vi "RunStatsForIndividualIpAddresses.vi"(8 "IpStatus (in)":T2[](array[typedef]) {"%rtk" scale=0.0..60.0; "TimePing" scale=0.0..60.0}, 11 "IP list (in)":T1) -> (0 "IpStatus(out)":T2[](array[typedef]) {"%rtk" scale=0.0..60.0; "TimePing" scale=0.0..60.0}, 3 "IP list (out)":T1)   [LabVIEW 2011]
uses:
  GPS String Capture Software/IP RTK status Indicator.ctl
  ArrayIpAddressesAndReportingCheckbox.ctl
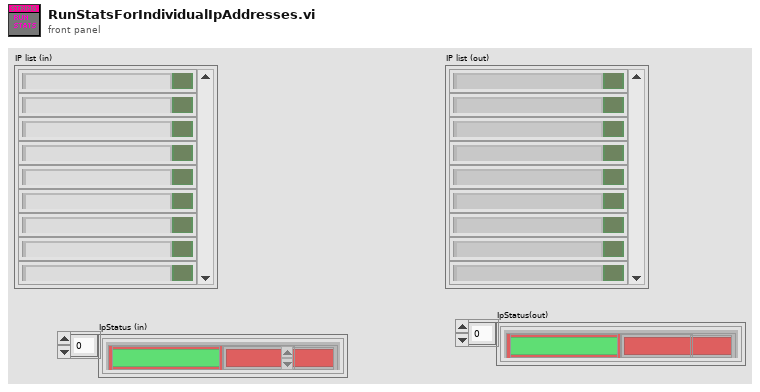
[diagram p1: front panel]
types:
  T1 = typedef "ArrayIpAddressesAndReportingCheckbox.ctl" = cluster{"IpAddress":string, "Report Errors":bool}[]
  T2 = typedef "IP RTK status Indicator.ctl" = cluster{"TimePing":dbl, "IP":string, "%rtk":dbl, "Lastrtk":string, "MinLastRTk":dbl, "RTK Count":bool[], "Last Nema Time":dbl, "Last RTK Time":dbl, "Last Ping time":dbl}
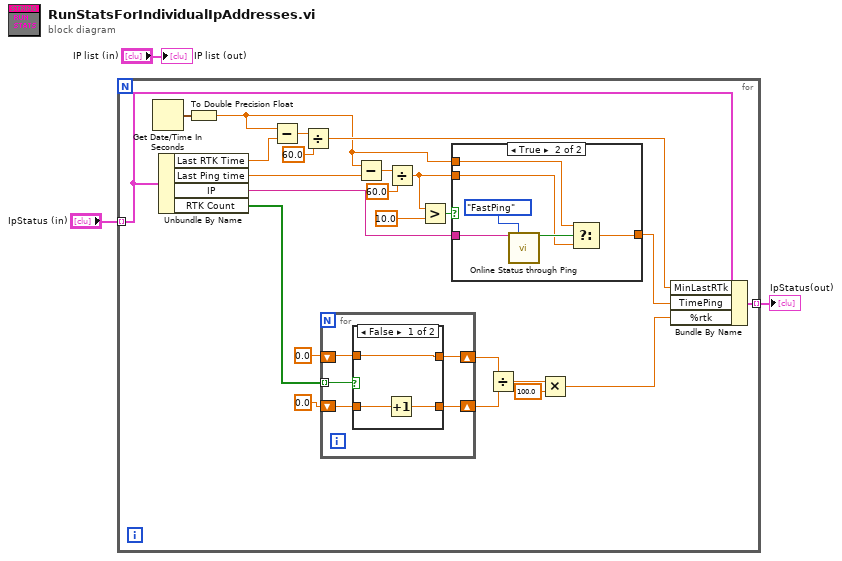
[diagram p0: block diagram]
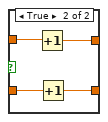
[diagram p2: hidden frame]
diagram:
  n1 = for {
    tunnel: "IpStatus (in)" -> [w20] mode=indexing
    tunnel: [w4] -> w2 mode=indexing
    n2 = Get Date/Time In Seconds() -> (seconds since 1Jan1904=w27:timestamp)
    n3 = Unbundle By Name(w20) -> ("Last RTK Time"=w26:dbl, "Last Ping time"=w21:dbl, "IP"=w14:string, "RTK Count"=w12:bool[])
    n4 = To Double Precision Float(number=w27) -> (double precision float=w13:dbl)
    n5 = Subtract(x=w13, y=w26) -> (x-y=w25:dbl)
    n6 = Divide(x=w25, y=60.0) -> (x/y=w19:dbl)
    n7 = for {
      tunnel: w12 -> [w32] mode=indexing
      shift-right: [w30] -> w9
      shift-left: 0.0 -> [w31]
      shift-right: [w28] -> w8
      shift-left: 0.0 -> [w29]
      n8 = case shown="False" w32 {
        tunnel: w31 -> [w35 w39]
        tunnel: [w35 w38] -> w30
        tunnel: w29 -> [w33 w37]
        tunnel: [w34 w36] -> w28
        frame False {
          n9 = Increment(x=w33) -> (x+1=w34:dbl)
        }
        frame True {
          n10 = Increment(x=w39) -> (x+1=w38:dbl)
          n11 = Increment(x=w37) -> (x+1=w36:dbl)
        }
      }
    }
    n12 = Subtract(x=w13, y=w21) -> (x-y=w22:dbl)
    n13 = Divide(x=w22, y=60.0) -> (x/y=w16:dbl)
    n14 = Greater?(x=w16, y=10.0) -> (0:w18:bool)
    n15 = case shown="True" w18 {
      tunnel: w16 -> [w40 w44]
      tunnel: [w40 w43] -> w15
      tunnel: w14 -> [_ w46]
      tunnel: w13 -> [_ w42]
      frame False {
      }
      frame True {
        n16 = call "Online Status through Ping.vi"("AddressToPing"=w46, "Ping Method"=enum16{"LongPing", "NormalPing", "FastPing"}."FastPing") -> ("Connection?"=w45:bool)  [unwired: 9 in, 4 out]
        n17 = Select(t=w42, s=w45, f=w44) -> (s? t:f=w43:dbl)
      }
    }
    n18 = Divide(x=w9, y=w8) -> (x/y=w7:dbl)
    n19 = Multiply(x=w7, y=100.0) -> (x*y=w5:dbl)
    n20 = Bundle By Name(cluster=w20, "MinLastRTk"=w19, "TimePing"=w15, "%rtk"=w5) -> (w4:T2)
  }
  "IpStatus(out)" <- w2
  "IP list (out)" <- "IP list (in)"
